vi "Wait 4 Move 2 Complete.vi"(8 "error in (no error)":errorcluster, 11 "Array":string[](array[string])) -> (0 "Error out":errorcluster)   [LabVIEW 2018]
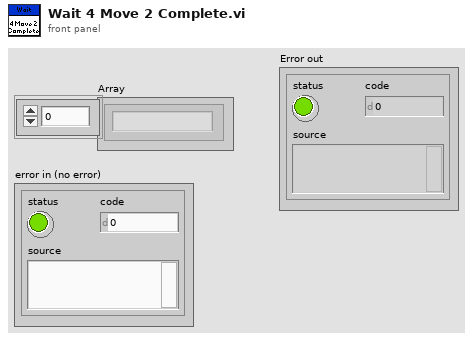
[diagram p1: front panel]
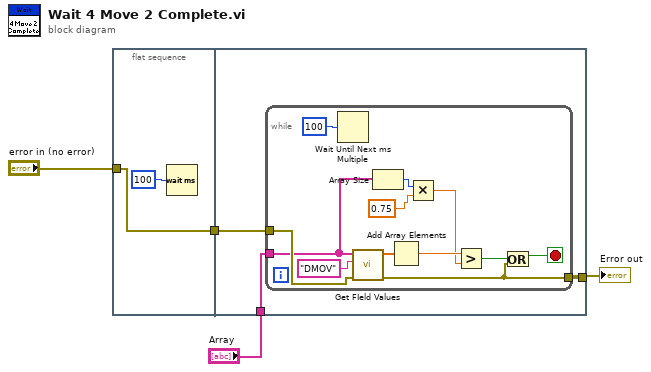
[diagram p0: block diagram]
diagram:
  n1 = flat-sequence {
    tunnel: "error in (no error)" -> [w5]
    tunnel: [w5] -> w2
    tunnel: "Array" -> [w9]
    tunnel: w2 -> [w8]
    tunnel: [w7] -> w1
    frame #0 {
      n2 = Wait (ms)(milliseconds to wait=u32 100) -> ()  [unwired: 1 out]
    }
    frame #1 {
      n3 = while {
        tunnel: w9 -> [w13]
        tunnel: w8 -> [w16]
        tunnel: [w14] -> w7
        stop <- w15 stop-if-true
        n4 = Wait Until Next ms Multiple(millisecond multiple=u32 100 ("milliseconds to wait")) -> ()  [unwired: 1 out]
        n5 = call "Get FIeld Values.vi"("Error in (no error)"=w16, "String"="DMOV", "Array in"=w13) -> ("Error out"=w14:errorcluster, "Array out"=w20:dbl[])  [unwired: 7 in]
        n6 = Array Size(array=w13) -> (size(s)=w12:i32)
        n7 = Add Array Elements(numeric array=w20) -> (sum=w19:dbl)
        n8 = Multiply(x=w12, y=0.75) -> (x*y=w10:dbl)
        n9 = Greater?(x=w19, y=w10) -> (0:w18:bool)
        n10 = Or(x=w18, y=w14) -> (x .or. y?=w15:bool)
      }
    }
  }
  "Error out" <- w1
